vi "Get Module Main Status.vi"(8 "error in":errorcluster, 10 "Library in":refnum<vi>, 11 "application Instance":refnum<vi>) -> (0 "error out":errorcluster, 1 "Module Exec State":T1(ring), 2 "Library Name":string)   [LabVIEW 2019, in "Panther Dashboard.lvlib"]
uses:
  Panther Dashboard.lvlib
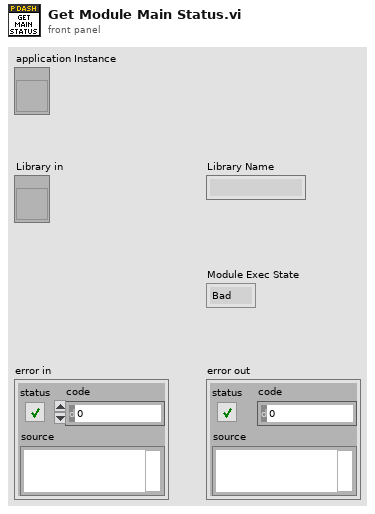
[diagram p1: front panel]
types:
  T1 = enum32{"Bad", "Idle", "Run top level", "Running"}
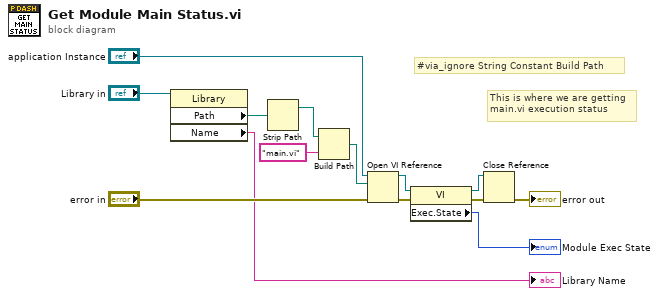
[diagram p0: block diagram]
diagram:
  # "#via_ignore String Constant Build Path"
  # "This is where we are getting\nmain.vi execution status"
  n1 = property class="Library"(reference="Library in") -> ("Path"=w4:path, "Name"=→"Library Name":string)  [unwired: 1 in, 2 out]
  n2 = Strip Path(path=w4) -> (stripped path=w5:path)  [unwired: 1 out]
  n3 = Build Path(base path=w5, name or relative path="main.vi" ("string")) -> (appended path=w7:path)
  n4 = Open VI Reference(application reference (local)="application Instance", vi path=w7, error in (no error)="error in") -> (vi reference=w8:refnum<vi>, error out=w14:errorcluster)  [unwired: 3 in]
  n5 = property class="VI"(reference=w8, error in=w14) -> (reference out=w9:refnum<vi>, error out=w13:errorcluster, "Exec.State"=→"Module Exec State":T1)
  n6 = Close Reference(reference=w9, error in (no error)=w13) -> (error out=→"error out":errorcluster)
